vi "JKI_Sprinkler.vi"() -> ()   [LabVIEW 2016]
doc: "The sprinkler controller simulates a lawn sprinkler control system that services four \nzones: North, South, East, and West. Controls on the front panel control the zone \nselection and simulate external conditions. Indicators on the front panel indicate the zone \nthat is currently being serviced and the elapsed time for that zone."
uses:
  Controls/Zone Setup.ctl
  Controls/Zone.ctl
  Controls/Zone Indicators.ctl
panel:
  out "Zone Indicators":T1 {"Timing" format="%#.2g"}
  out "Controller Status":string
  in  "Simulation Controls":T2 {"Water Pressure Sensor (%)" scale=0.0..100.0}
  in  "Zone Setup Array":T3[](array[typedef])
  in  "Controls":T5
  # "Rain"
  # "No Rain"
  # "Continuous"
  # "Single"
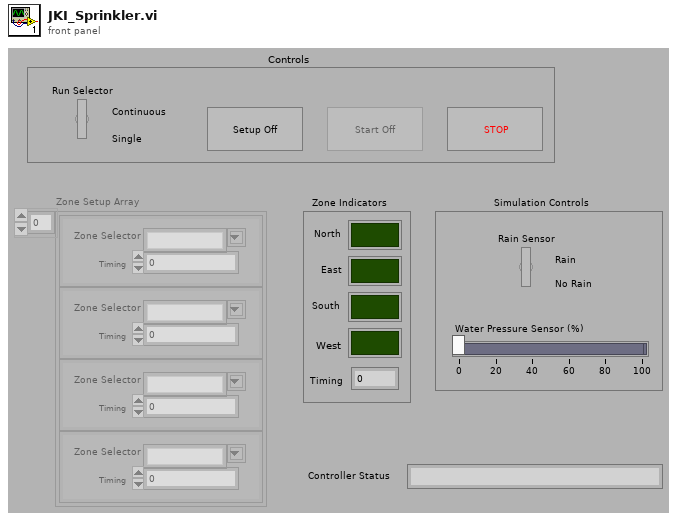
[diagram p1: front panel]
types:
  T1 = typedef "Zone Indicators.ctl" = cluster{"North":bool, "East":bool, "South":bool, "West":bool, "Timing":dbl}
  T2 = cluster{"Rain Sensor":bool, "Water Pressure Sensor (%)":dbl}
  T3 = typedef "Zone Setup.ctl" = cluster{"Zone Selector":T4, "Timing":u32}
  T4 = typedef "Zone.ctl" = string
  T5 = cluster{"Run Selector":bool, "Setup":bool, "Start":bool, "Stop":bool}
  T6 = enum32{"invalid app kind", "Development System", "Run Time System", "Student Edition", "Embedded LabVIEW", "Evaluation", "Custom"}
  T7 = enum8{"Enabled", "Disabled", "Disabled and Grayed Out"}
  T8 = enum32{"Invalid", "Standard", "Closed", "Hidden", "Minimized", "Maximized"}
  T9 = cluster{"Core":cluster{"Current VI Reference":refnum<vi>, "Close Panel on Exit?":bool}, "Your boolean":bool, "Your string data":string, "Index Zone":i32}
  T10 = cluster{"Current VI Reference":refnum<vi>, "Close Panel on Exit?":bool}
  T11 = enum16{"Always On", "Always Off", "Off While Running"}
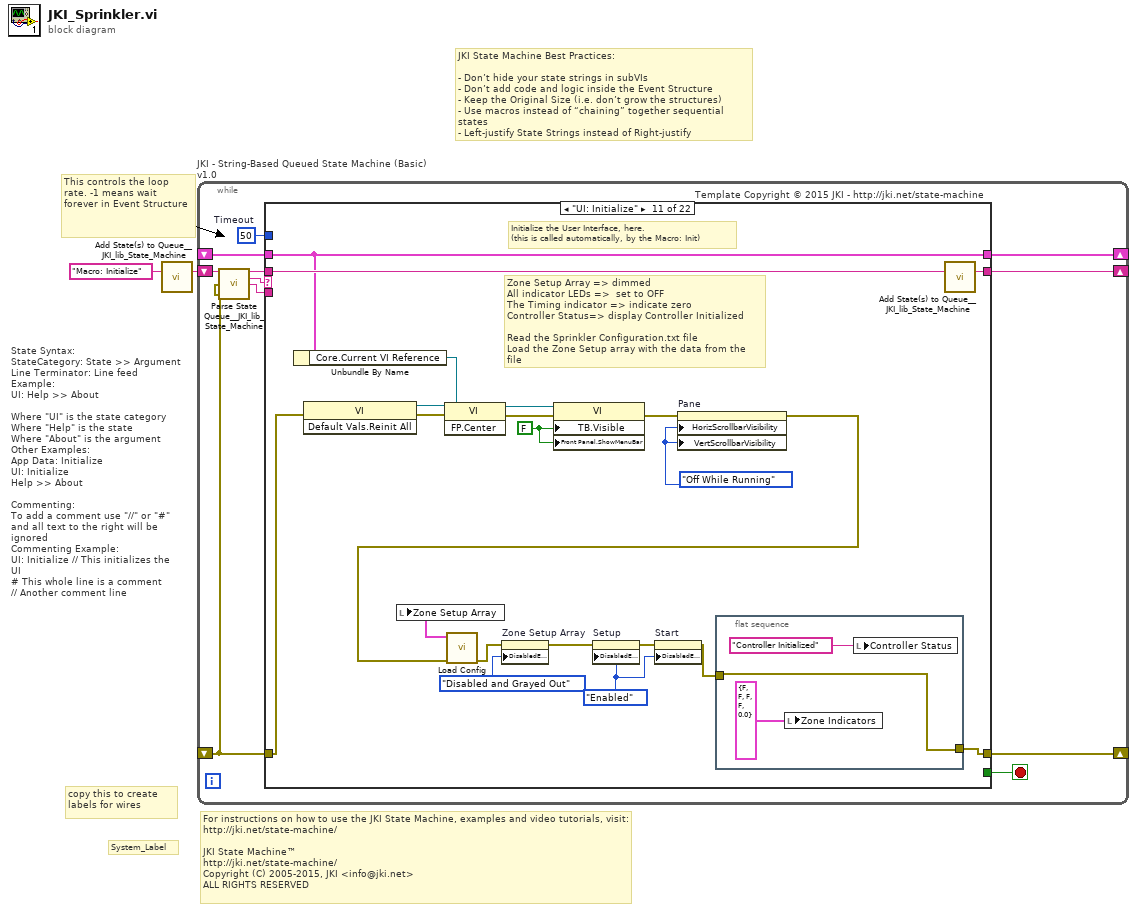
[diagram p0: block diagram]
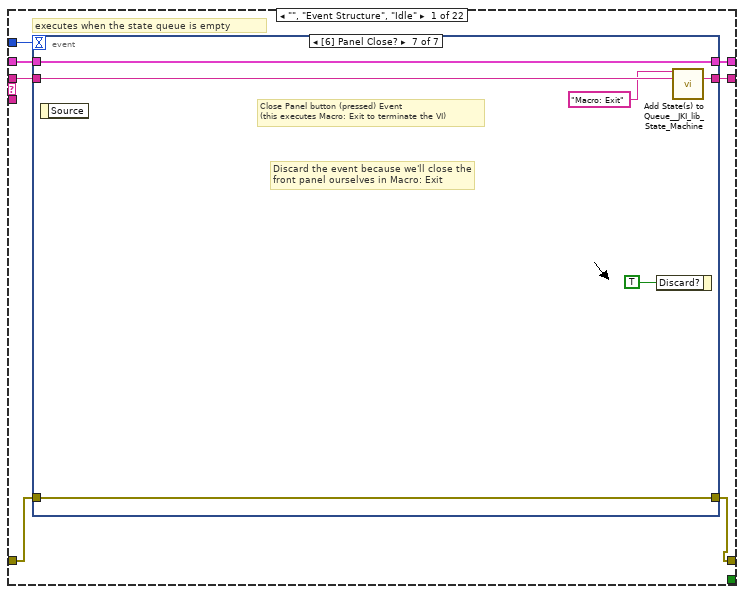
[diagram p2: hidden frame]
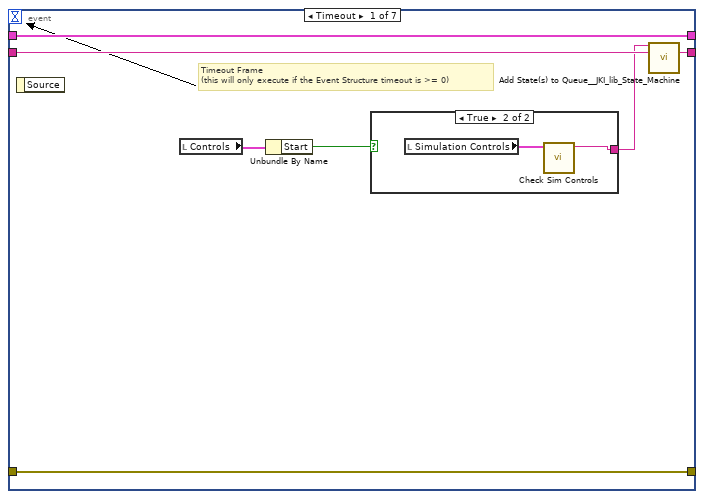
[diagram p3: hidden frame]
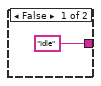
[diagram p4: hidden frame]
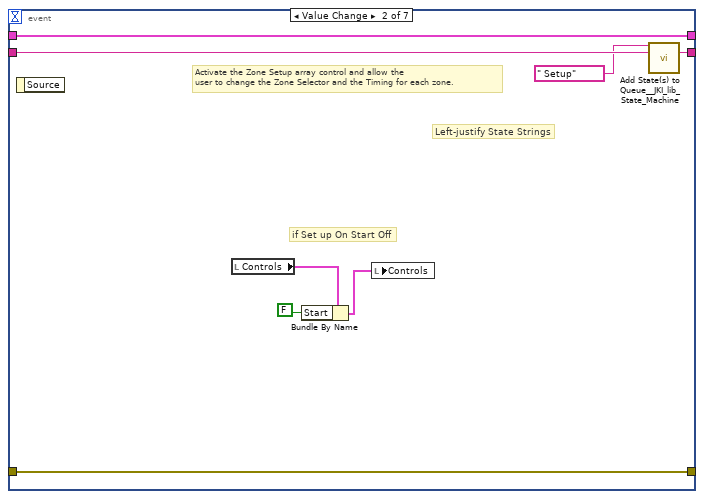
[diagram p5: hidden frame]
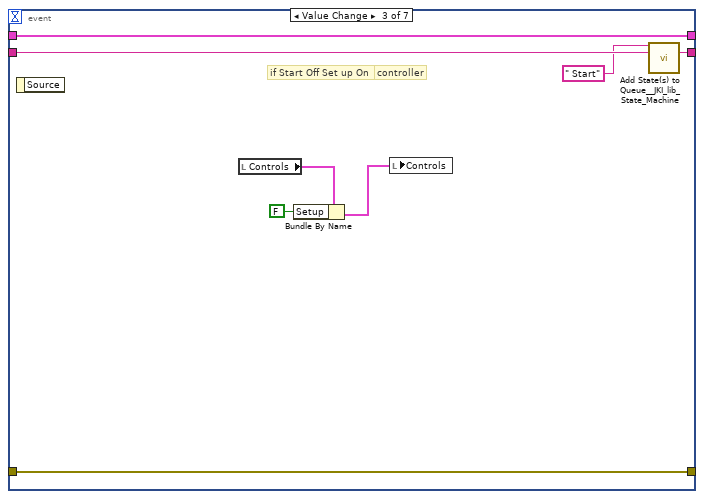
[diagram p6: hidden frame]
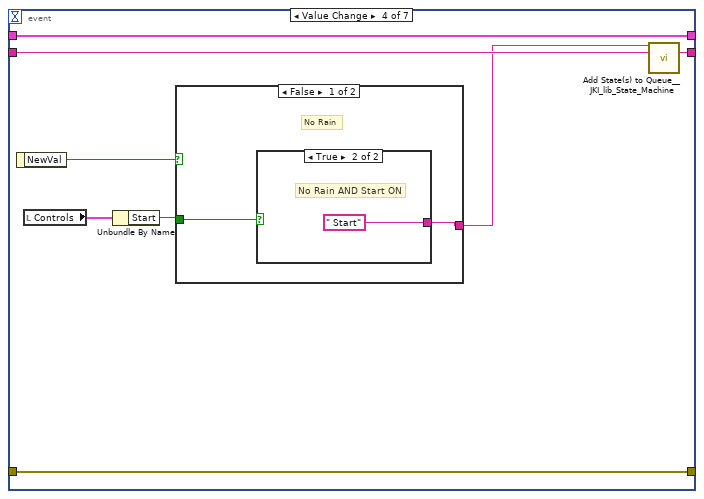
[diagram p7: hidden frame]
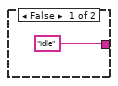
[diagram p8: hidden frame]
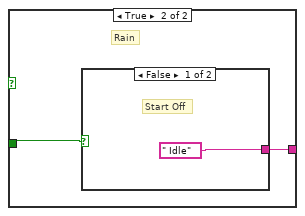
[diagram p9: hidden frame]
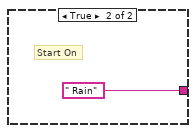
[diagram p10: hidden frame]
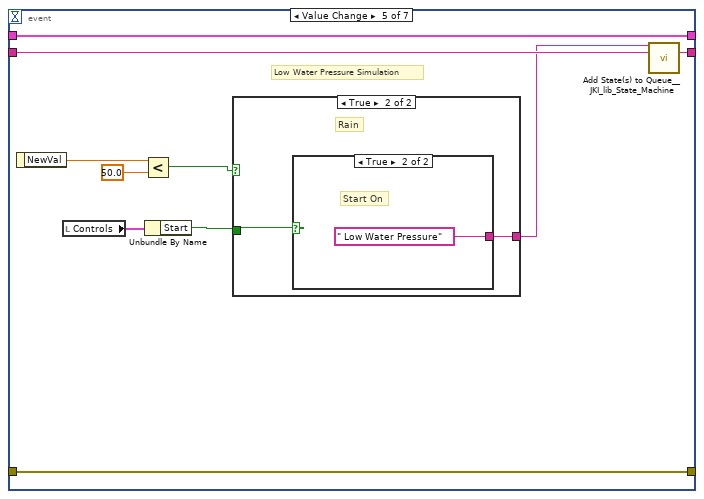
[diagram p11: hidden frame]
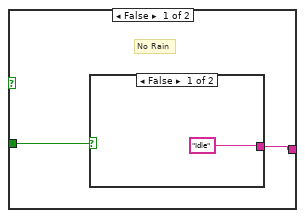
[diagram p12: hidden frame]
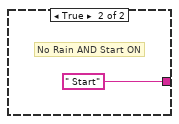
[diagram p13: hidden frame]
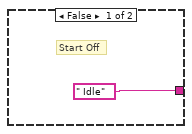
[diagram p14: hidden frame]
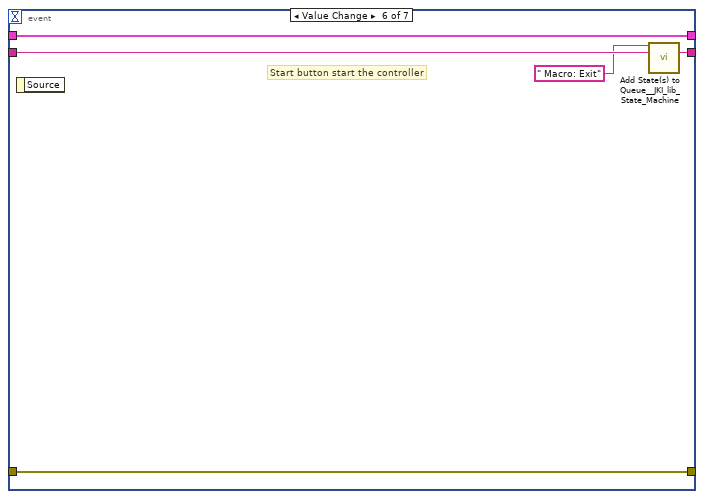
[diagram p15: hidden frame]
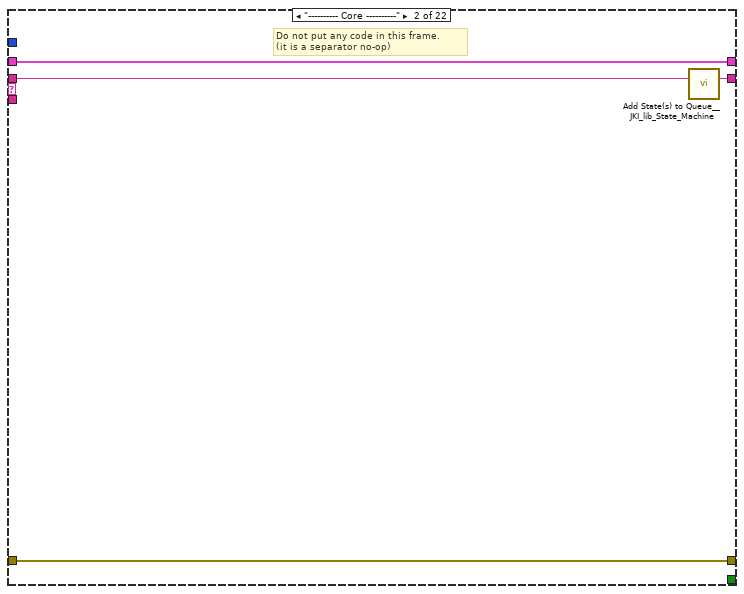
[diagram p16: hidden frame]
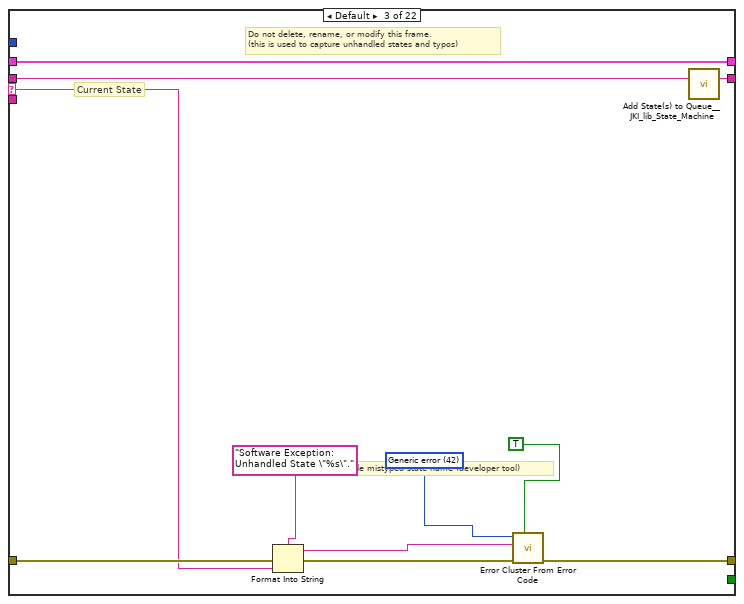
[diagram p17: hidden frame]
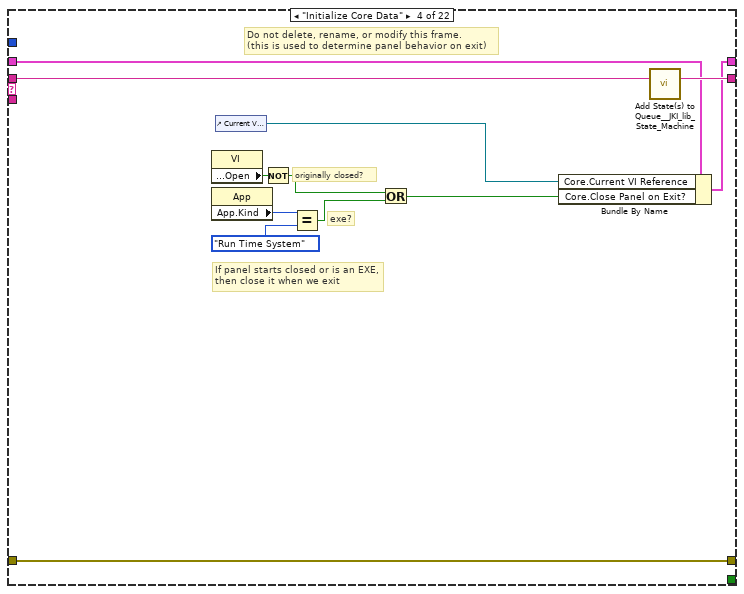
[diagram p18: hidden frame]
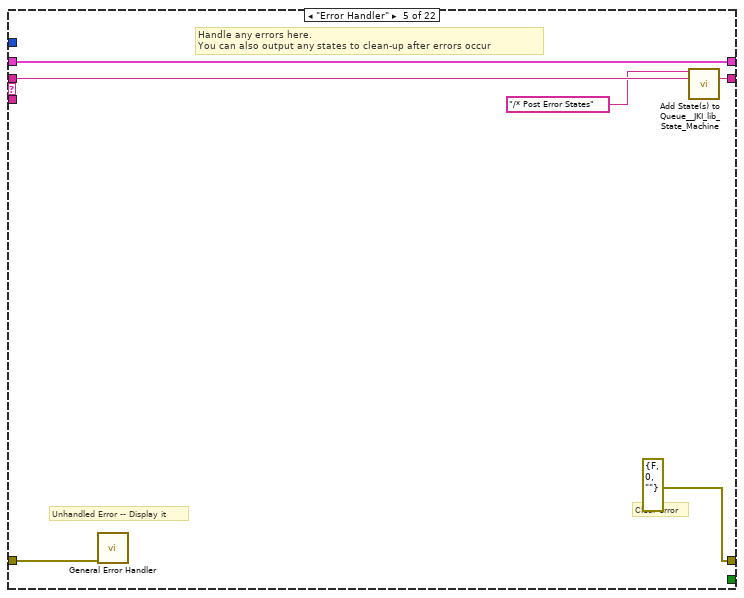
[diagram p19: hidden frame]
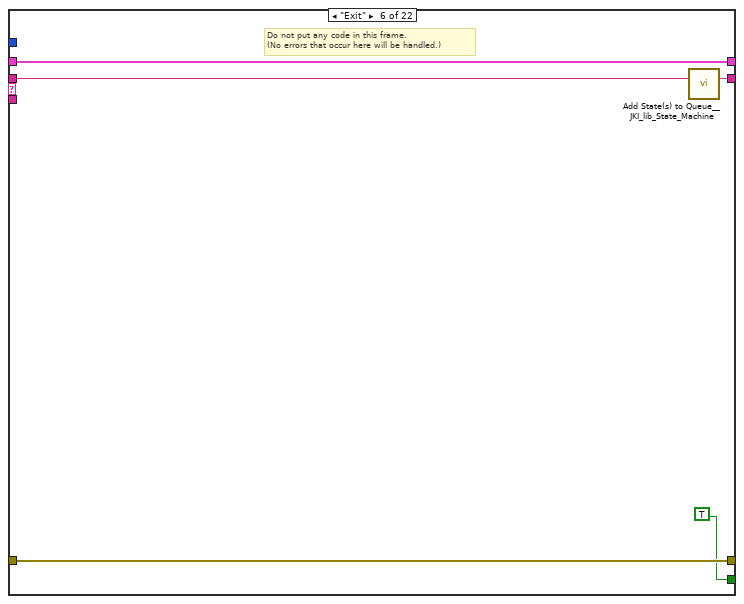
[diagram p20: hidden frame]
diagram:
  # "JKI State Machine Best Practices:\n\n- Don’t hide your state strings in subVIs\n- Don’t add code and logic inside the Event Structure\n- Keep the Original Size (i.e. don’t grow the structures)\n- Use macros instead of “chaining” together sequential states\n- Left-justify State Strings instead of Right-justify"
  # "For instructions on how to use the JKI State Machine, examples and video tutorials, visit:\nhttp://jki.net/state-machine/\n\nJKI State Machine™\nhttp://jki.net/state-machine/\nCopyright (C) 2005-2015, JKI <info@jki.net>\nALL RIGHTS RESERVED"
  # "State Syntax:\nStateCategory: State >> Argument\nLine Terminator: Line feed\nExample:\nUI: Help >> About\n\nWhere \"UI\" is the state category\nWhere \"Help\" is the state\nWhere \"About\" is the argument\nOther Examples:\nApp Data: Initialize\nUI: Initialize\nHelp >> About\n\nCommenting:\nTo add a comment use \"//\" or \"#\" and all text to the right will be ignored\nCommenting Example:\nUI: Initialize // This initializes the UI\n# This whole line is a comment\n// Another comment line"
  # "copy this to create labels for wires"
  # "This controls the loop rate. -1 means wait forever in Event Structure"
  # "System_Label"
  n1 = call <vilib>:"Add State(s) to Queue__JKI_lib_State_Machine.vi"("State(s) in (\"\")"="Macro: Initialize") -> ("States Out"=w2:string)  [unwired: 14 in]
  n2 = while "JKI - String-Based Queued State Machine (Basic) v1.0" {
    shift-right: [w6] -> _
    shift-left: _ -> [w5]
    shift-right: [w9] -> _
    shift-left: _ -> [w3]
    shift-right: [w8] -> _
    shift-left: w2 -> [w10]
    stop <- w7 stop-if-true
    w4 = 50  # Timeout
    # "Template Copyright © 2015 JKI - http://jki.net/state-machine"
    n3 = call <vilib>:"Parse State Queue__JKI_lib_State_Machine.vi"("State Queue"=w10, "Error In (no error)"=w3) -> ("Remaining States"=w12:string, "Current State"=w13:string, "Arguments"=w11:string)  [unwired: 11 in]
    n4 = case shown="\"UI: Initialize\"" w13 {
      selector: w13 -> [_ _ w96 _ _ _ _ _ _ _ _ _ _ _ _ _ _ _ _ _ _ _]
      tunnel: w12 -> [w20 w95 w100 w118 w124 w129 w133 w141 w147 w151 w171 w180 w191 w217 w222 w233 w237 w248 w264 w270 w276 w290]
      tunnel: w11 -> [_ _ _ _ _ _ _ _ _ _ _ w175 w185 _ _ _ _ _ _ _ _ _]
      tunnel: w5 -> [w18 w92 w98 w109 w121 w127 w130 _ w142 w148 w167 w178 w187 w214 w219 w230 w234 w246 w258 w268 w274 w286]
      tunnel: [w17 w93 w102 w115 errorcluster {"status"=FALSE, "code"=0, "source"=""} ("error out") w126 w131 w138 w143 w149 w153 w176 w188 w215 w220 w231 w235 w243 w260 w266 w272 w279] -> w9
      tunnel: w3 -> [w16 w93 w101 w115 w120 w126 w131 w138 w144 w149 w163 w177 w189 w215 w220 w231 w235 w245 w261 w266 w272 w281]
      tunnel: [w19 w94 w99 w117 w123 w128 w132 w140 w146 w150 w170 w179 w190 w216 w221 w232 w236 w247 w263 w269 w275 w289] -> w8
      tunnel: [_ _ _ _ _ TRUE _ _ _ _ _ _ _ _ _ _ _ _ _ _ _ _] -> w7
      tunnel: [w15 w92 w98 w116 w121 w127 w130 w139 w142 w148 w167 w178 w187 w214 w219 w230 w234 w246 w257 w268 w274 w287] -> w6
      tunnel: w4 -> [w14 _ _ _ _ _ _ _ _ _ _ _ _ _ _ _ _ _ _ _ _ _]
      frame "", "Event Structure", "Idle" {
        # "executes when the state queue is empty"
        n5 = event shown="[6] Panel Close?" {
          selector: _ -> [_ _ _ _ _ _ _]
          dyn-events: _ -> [_ _ _ _ _ _ _]
          timeout: w14 -> [_ _ _ _ _ _ _]
          tunnel: w20 -> [w27 w38 w46 w54 w72 w85 w91]
          tunnel: [w26 w37 w45 w53 w71 w84 w90] -> w19
          tunnel: w18 -> [w24 w35 w43 w51 w69 w82 w88]
          tunnel: [w25 w36 w44 w52 w70 w83 w89] -> w17
          tunnel: w16 -> [w25 w36 w44 w52 w70 w83 w89]
          tunnel: [w24 w35 w43 w51 w69 w82 w88] -> w15
          event Timeout {
            # "Timeout Frame\n(this will only execute if the Event Structure timeout is >= 0)"
            n6 = event-data() -> ()  [unwired: 1 in, 1 out]
            n7 = local read "Controls"() -> (w23:T5)
            n8 = Unbundle By Name(w23) -> ("Start"=w21:bool)
            n9 = case shown="True" w21 {
              tunnel: ["Idle" w29] -> w22
              frame False {
              }
              frame True {
                n10 = local read "Simulation Controls"() -> (w30:T2)
                n11 = call "Check Sim Controls.vi"("Simulation Controls"=w30) -> ("State"=w29:string)  [unwired: 9 in, 1 out]
              }
            }
            n12 = call <vilib>:"Add State(s) to Queue__JKI_lib_State_Machine.vi"("State(s) in Front (\"\")"=w22, "State(s) in (\"\")"=w27) -> ("States Out"=w26:string)  [unwired: 13 in]
          }
          event "Controls.Setup": Value Change {
            # "if Set up On Start Off"
            # "Left-justify State Strings"
            # "Activate the Zone Setup array control and allow the \nuser to change the Zone Selector and the Timing for each zone."
            n13 = event-data() -> ()  [unwired: 1 in, 1 out]
            n14 = local read "Controls"() -> (w33:T5)
            n15 = Bundle By Name(cluster=w33, "Start"=FALSE) -> (w32:T5)
            n16 = local write "Controls"(w32) -> ()
            n17 = call <vilib>:"Add State(s) to Queue__JKI_lib_State_Machine.vi"("State(s) in Front (\"\")"=" Setup", "State(s) in (\"\")"=w38) -> ("States Out"=w37:string)  [unwired: 13 in]
          }
          event "Controls.Start": Value Change {
            # "if Start Off Set up On"
            # "Start button start the controller"
            n18 = event-data() -> ()  [unwired: 1 in, 1 out]
            n19 = local read "Controls"() -> (w41:T5)
            n20 = Bundle By Name(cluster=w41, "Setup"=FALSE) -> (w40:T5)
            n21 = local write "Controls"(w40) -> ()
            n22 = call <vilib>:"Add State(s) to Queue__JKI_lib_State_Machine.vi"("State(s) in Front (\"\")"=" Start", "State(s) in (\"\")"=w46) -> ("States Out"=w45:string)  [unwired: 13 in]
          }
          event "Simulation Controls.Rain Sensor": Value Change {
            n23 = event-data() -> ("NewVal"=w50:bool)  [unwired: 1 in]
            n24 = local read "Controls"() -> (w49:T5)
            n25 = Unbundle By Name(w49) -> ("Start"=w48:bool)
            n26 = case shown="False" w50 {
              tunnel: w48 -> [w56 w60]
              tunnel: [w55 w59] -> w47
              frame False {
                # "No Rain"
                n27 = case shown="True" w56 {
                  tunnel: ["Idle" " Start"] -> w55
                  frame False {
                  }
                  frame True {
                    # "No Rain AND Start ON"
                  }
                }
              }
              frame True {
                # "Rain"
                n28 = case shown="False" w60 {
                  tunnel: [" Idle" " Rain"] -> w59
                  frame False {
                    # "Start Off"
                  }
                  frame True {
                    # "Start On"
                  }
                }
              }
            }
            n29 = call <vilib>:"Add State(s) to Queue__JKI_lib_State_Machine.vi"("State(s) in Front (\"\")"=w47, "State(s) in (\"\")"=w54) -> ("States Out"=w53:string)  [unwired: 13 in]
          }
          event "Simulation Controls.Water Pressure Sensor (%)": Value Change {
            # "Low Water Pressure Simulation"
            n30 = event-data() -> ("NewVal"=w68:dbl)  [unwired: 1 in]
            n31 = local read "Controls"() -> (w66:T5)
            n32 = Less?(x=w68, y=50.0) -> (x < y?=w64:bool)
            n33 = Unbundle By Name(w66) -> ("Start"=w65:bool)
            n34 = case shown="True" w64 {
              tunnel: w65 -> [w74 w78]
              tunnel: [w73 w77] -> w63
              frame False {
                # "No Rain"
                n35 = case shown="False" w74 {
                  tunnel: ["Idle" " Start"] -> w73
                  frame False {
                  }
                  frame True {
                    # "No Rain AND Start ON"
                  }
                }
              }
              frame True {
                # "Rain"
                n36 = case shown="True" w78 {
                  tunnel: [" Idle" " Low Water Pressure"] -> w77
                  frame False {
                    # "Start Off"
                  }
                  frame True {
                    # "Start On"
                  }
                }
              }
            }
            n37 = call <vilib>:"Add State(s) to Queue__JKI_lib_State_Machine.vi"("State(s) in Front (\"\")"=w63, "State(s) in (\"\")"=w72) -> ("States Out"=w71:string)  [unwired: 13 in]
          }
          event "Controls.Stop": Value Change {
            # "Start button start the controller"
            n38 = event-data() -> ()  [unwired: 1 in, 1 out]
            n39 = call <vilib>:"Add State(s) to Queue__JKI_lib_State_Machine.vi"("State(s) in Front (\"\")"=" Macro: Exit", "State(s) in (\"\")"=w85) -> ("States Out"=w84:string)  [unwired: 13 in]
          }
          event Panel Close? {
            # "Discard the event because we'll close the front panel ourselves in Macro: Exit"
            # "Close Panel button (pressed) Event\n(this executes Macro: Exit to terminate the VI)"
            n40 = event-data() -> ()  [unwired: 1 in, 1 out]
            n41 = event-data("Discard?"=TRUE) -> ()  [unwired: 1 in, 1 out]
            n42 = call <vilib>:"Add State(s) to Queue__JKI_lib_State_Machine.vi"("State(s) in Front (\"\")"="Macro: Exit", "State(s) in (\"\")"=w91) -> ("States Out"=w90:string)  [unwired: 13 in]
          }
        }
      }
      frame "---------- Core ----------" {
        # "Do not put any code in this frame.\n(it is a separator no-op)"
        n43 = call <vilib>:"Add State(s) to Queue__JKI_lib_State_Machine.vi"("State(s) in (\"\")"=w95) -> ("States Out"=w94:string)  [unwired: 14 in]
      }
      frame Default {
        w105 = 42 items=["No error", "Argument error", "Memory is full", "Out of zone", "End of file", "File already open", "Generic file I/O error", "File not found", "File permission error", "Disk is full", "Duplicate path", "Too many files open", "System feature not enabled", "Resource file not found", "Cannot add resource", "Resource not found", "Image not found", "Image memory error", "Pen does not exist", "Config type invalid", "Config token not found", "Config parse error", "Config memory error", "Bad external code format", "Bad external code offset", "External code not present", "Null window", "Destroy window error", "Null menu", "Print aborted", "Bad print record", "Print driver error", "Windows error during printing", "Memory error during printing", "Print dialog error", "Generic print error", "Invalid device refnum", "Device not found", "Device parameter error", "Device unit error", "Cannot open device", "Device call aborted", "Generic error", "Cancelled by user", "Object ID too low", "Object ID too high", "Object not in heap", "Unknown heap", "Unknown object (invalid DefProc)", "Unknown object (DefProc not in table)", "Message out of range", "Invalid (null) method", "Unknown message", "Manager call not supported", "Bad address", "Network operation in progress", "Network operation timed out", "Connection is busy", "Network attribute not supported", "Network error", "Address in use", "System out of memory", "Connection aborted", "Connection refused", "Not connected", "Already connected", "Connection closed", "Initialization error (interapplication manager)", "Bad occurrence", "Wait on unbound occurrence handler", "Occurrence queue overflow", "Datalog type conflict", "Unused", "Unrecognized type (interapplication manager)", "Memory corrupt", "Failed to make temporary DLL", "Old CIN version", "Drag socket not found", "Failed to load drop-object", "Failed to register OLE object", "Failed to release OLE object", "Format specifier type mismatch", "Unknown format specifier", "Too few format specifiers", "Too many format specifiers", "Scan failed", "Newer CIN version", "Error converting to variant", "Runtime menu error", "Password tampered", "Variant attribute not found", "Incompatible variant data type", "Event data is not available", "Event Store is not present", "Occurrence is not found", "Event Queue is not created", "Event info is not available", "Refnum passed is NULL", "Error retrieving Class GUID", "Error retrieving CoClass GUID", "Error retrieving TypeLib GUID.", "Bad built application magic bytes.", "Specific driver is different from the specific driver associated with the Logical Name.", "There is no session opened to the class driver.", "Max Error", "MAX - Error with config objects", "MAX - Error loading configuration", "MAX - Group not supported"]
        # "Current State"
        # "Do not delete, rename, or modify this frame.\n(this is used to capture unhandled states and typos)"
        # "Handle mistyped state name (developer tool)"
        n44 = Format Into String(format string="Software Exception: Unhandled State \"%s\"." ("message"), error in=w101, w96) -> (resulting string=w104:string, error out=w103:errorcluster)  [unwired: 1 in]
        n45 = call <vilib>:"Error Cluster From Error Code.vi"("show call chain? (False)"=TRUE, "error in (no error)"=w103, "error message (\"\")"=w104, "error code (0)"=w105) -> ("error out"=w102:errorcluster)  [unwired: 5 in]
        n46 = call <vilib>:"Add State(s) to Queue__JKI_lib_State_Machine.vi"("State(s) in (\"\")"=w100) -> ("States Out"=w99:string)  [unwired: 14 in]
      }
      frame "Initialize Core Data" {
        # "Do not delete, rename, or modify this frame.\n(this is used to determine panel behavior on exit)"
        # "originally closed?"
        # "exe?"
        # "If panel starts closed or is an EXE, then close it when we exit"
        n47 = property class="VI"() -> ("Front Panel.Open"=w114:bool)  [unwired: 2 in, 2 out]
        n48 = property class="App"() -> ("App.Kind"=w113:T6)  [unwired: 2 in, 2 out]
        n49 = control-ref of="Current VI Reference"() -> (w107:refnum<vi>)
        n50 = Not(x=w114) -> (.not. x?=w111:bool)
        n51 = Equal?(x=w113, y=T6."Run Time System" ("Application:Kind")) -> (x = y?=w110:bool)
        n52 = Or(x=w111, y=w110) -> (x .or. y?=w108:bool)
        n53 = Bundle By Name(cluster=w109, "Core.Current VI Reference"=w107, "Core.Close Panel on Exit?"=w108) -> (w116:T9)
        n54 = call <vilib>:"Add State(s) to Queue__JKI_lib_State_Machine.vi"("State(s) in (\"\")"=w118) -> ("States Out"=w117:string)  [unwired: 14 in]
      }
      frame "Error Handler" {
        # "Unhandled Error -- Display it"
        # "Handle any errors here.\nYou can also output any states to clean-up after errors occur"
        # "Clear error"
        n55 = call <vilib>:"General Error Handler.vi"("error in (no error)"=w120) -> ()  [unwired: 10 in, 5 out]
        n56 = call <vilib>:"Add State(s) to Queue__JKI_lib_State_Machine.vi"("State(s) in Front (\"\")"="/* Post Error States", "State(s) in (\"\")"=w124) -> ("States Out"=w123:string)  [unwired: 13 in]
      }
      frame "Exit" {
        # "Do not put any code in this frame.\n(No errors that occur here will be handled.)"
        n57 = call <vilib>:"Add State(s) to Queue__JKI_lib_State_Machine.vi"("State(s) in (\"\")"=w129) -> ("States Out"=w128:string)  [unwired: 14 in]
      }
      frame "---------- Data ----------" {
        # "Do not put any code in this frame.\n(It is a separator no-op. You can make a copy of this frame to create a new Data frame)"
        n58 = call <vilib>:"Add State(s) to Queue__JKI_lib_State_Machine.vi"("State(s) in (\"\")"=w133) -> ("States Out"=w132:string)  [unwired: 14 in]
      }
      frame "Data: Initialize" {
        w134 = TRUE  # Your boolean
        w135 = 0  # Index Zone
        w136 = T10 {"Current VI Reference"=refnum, "Close Panel on Exit?"=FALSE}  # Core
        w137 = ""  # Your string data
        # "do not delete - used by framework"
        # "Expand Bundle to add new data elements to shift register data."
        # "Data names and types of shift register data are defined by this bundle."
        # "Initialize the shift-register data, here.\n(data names are defined by what you wire into the bundle function)"
        n59 = Bundle("Core"=w136, "Your boolean"=w134, "Your string data"=w137, "Index Zone"=w135) -> (w139:T9)  [unwired: 1 in]
        n60 = call <vilib>:"Add State(s) to Queue__JKI_lib_State_Machine.vi"("State(s) in (\"\")"=w141) -> ("States Out"=w140:string)  [unwired: 14 in]
      }
      frame "Data: Cleanup" {
        # "Cleanup any data and references, here.\n(this is called automatically, by the Macro: Exit)"
        n61 = Unbundle By Name(w142) -> ("Core.Current VI Reference"=w145:refnum<vi>)
        n62 = Close Reference(reference=w145, error in (no error)=w144) -> (error out=w143:errorcluster)
        n63 = call <vilib>:"Add State(s) to Queue__JKI_lib_State_Machine.vi"("State(s) in (\"\")"=w147) -> ("States Out"=w146:string)  [unwired: 14 in]
      }
      frame "---------- UI ----------" {
        # "Do not put any code in this frame.\n(It is a separator no-op. You can make a copy of this frame to create a new UI frame)"
        n64 = call <vilib>:"Add State(s) to Queue__JKI_lib_State_Machine.vi"("State(s) in (\"\")"=w151) -> ("States Out"=w150:string)  [unwired: 14 in]
      }
      frame "UI: Initialize" {
        w152 = T11."Off While Running" ("Horizontal Scrollbar Visibility")
        w164 = FALSE ("Tool Bar:Visible")
        w156 = T7."Enabled" ("Disabled")
        # "Zone Setup Array => dimmed \nAll indicator LEDs =>  set to OFF \nThe Timing indicator => indicate zero  \nController Status=> display Controller Initialized\n\nRead the Sprinkler Configuration.txt file\nLoad the Zone Setup array with the data from the file"
        # "Initialize the User Interface, here.\n(this is called automatically, by the Macro: Init)"
        n65 = Unbundle By Name(w167) -> ("Core.Current VI Reference"=w166:refnum<vi>)
        n66 = invoke class="VI" method="Default Vals.Reinit All"(reference=w166, error in=w163) -> (error out=w162:errorcluster)  [unwired: 1 in, 2 out]
        n67 = invoke class="VI" method="FP.Center"(reference=w166, error in=w162) -> (reference out=w165:refnum<vi>, error out=w161:errorcluster)  [unwired: 1 in, 1 out]
        n68 = property class="VI"(reference=w165, error in=w161, "TB.Visible"=w164, "Front Panel.ShowMenuBar"=w164) -> (error out=w160:errorcluster)  [unwired: 1 out]
        n69 = property on="Pane" class="Pane"(error in=w160, "HorizScrollbarVisibility"=w152, "VertScrollbarVisibility"=w152) -> (error out=w159:errorcluster)  [unwired: 1 in, 1 out]
        n70 = call "Load Config.vi"("error in"=w159) -> ("error out"=w158:errorcluster, "Zone Setup Array"=w168:T3[])  [unwired: 9 in]
        n71 = local write "Zone Setup Array"(w168) -> ()
        n72 = property on="Zone Setup Array" class="Arr (strict)"(error in=w158, "DisabledEnum"=T7."Disabled and Grayed Out" ("Disabled")) -> (error out=w157:errorcluster)  [unwired: 1 in, 1 out]
        n73 = property on="Setup" class="Bool (strict)"(error in=w157, "DisabledEnum"=w156) -> (error out=w155:errorcluster)  [unwired: 1 in, 1 out]
        n74 = property on="Start" class="Bool (strict)"(error in=w155, "DisabledEnum"=w156) -> (error out=w154:errorcluster)  [unwired: 1 in, 1 out]
        n75 = flat-sequence {
          tunnel: w154 -> [w172]
          tunnel: [w172] -> w153
          frame #0 {
            n76 = local write "Zone Indicators"(T1 {"North"=FALSE, "East"=FALSE, "South"=FALSE, "West"=FALSE, "Timing"=0.0} ("Zone Indicators")) -> ()
            n77 = local write "Controller Status"("Controller Initialized") -> ()
          }
        }
        n78 = call <vilib>:"Add State(s) to Queue__JKI_lib_State_Machine.vi"("State(s) in (\"\")"=w171) -> ("States Out"=w170:string)  [unwired: 14 in]
      }
      frame "UI: Cursor Set" {
        # "Argument"
        # "Set and Unset Cursor Busy.\n(Usage: \"UI: Cursor Set >> Busy|Idle\")"
        n79 = case shown="\"Idle\", Default" w175 {
          tunnel: w177 -> [w182 w184]
          tunnel: [w181 w183] -> w176
          frame "Idle", Default {
            n80 = call <vilib>:"Unset Busy.vi"("error in (no error)"=w182) -> ("error out"=w181:errorcluster)  [unwired: 10 in]
          }
          frame "Busy" {
            n81 = call <vilib>:"Set Busy.vi"("error in (no error)"=w184) -> ("error out"=w183:errorcluster)  [unwired: 9 in, 1 out]
          }
        }
        n82 = call <vilib>:"Add State(s) to Queue__JKI_lib_State_Machine.vi"("State(s) in (\"\")"=w180) -> ("States Out"=w179:string)  [unwired: 14 in]
      }
      frame "UI: Front Panel State" {
        # "Argument"
        # "Set Front Panel Open or Closed\n(Usage: \"UI: Front Panel State >> Open|Close\")"
        n83 = Unbundle By Name(w187) -> ("Core.Current VI Reference"=w186:refnum<vi>)
        n84 = case shown="\"Open\", Default" w185 {
          tunnel: w189 -> [w195 w208]
          tunnel: [w197 w209] -> w188
          tunnel: w186 -> [w196 w206]
          frame "Open", Default {
            n85 = property class="VI"(reference=w196, error in=w195) -> (reference out=w193:refnum<vi>, error out=w194:errorcluster, "Front Panel.Open"=w192:bool)
            n86 = case shown="True" w192 {
              tunnel: [w200 w203] -> w197
              tunnel: w194 -> [w199 w203]
              tunnel: w193 -> [w198 _]
              frame False {
                n87 = invoke class="VI" method="FP.Open"(reference=w198, error in=w199, "Activate"=TRUE, "State"=T8."Standard") -> (error out=w200:errorcluster)  [unwired: 1 in, 4 out]
              }
              frame True {
              }
            }
          }
          frame "Close" {
            n88 = property class="VI"(reference=w206, error in=w208) -> (reference out=w205:refnum<vi>, error out=w207:errorcluster, "Front Panel.Open"=w204:bool)
            n89 = case shown="True" w204 {
              tunnel: [w210 w213] -> w209
              tunnel: w207 -> [w210 w212]
              tunnel: w205 -> [_ w211]
              frame False {
              }
              frame True {
                n90 = invoke class="VI" method="FP.Close"(reference=w211, error in=w212) -> (error out=w213:errorcluster)  [unwired: 1 in, 2 out]
              }
            }
          }
        }
        n91 = call <vilib>:"Add State(s) to Queue__JKI_lib_State_Machine.vi"("State(s) in (\"\")"=w191) -> ("States Out"=w190:string)  [unwired: 14 in]
      }
      frame "---------- Macro ----------" {
        # "Do not put any code in this frame.\n(It is a separator no-op. You can make a copy of this frame to create a new Macro frame)"
        n92 = call <vilib>:"Add State(s) to Queue__JKI_lib_State_Machine.vi"("State(s) in (\"\")"=w217) -> ("States Out"=w216:string)  [unwired: 14 in]
      }
      frame "Macro: Initialize" {
        w218 = "Data: Initialize\nInitialize Core Data\nUI: Initialize\nUI: Front Panel State >> Open"  # Data: Initialize Initialize Core Data UI: Initialize UI: Front Panel State >> Open
        # "Initialization Macro\n(This is called once, when the VI starts)"
        n93 = call <vilib>:"Add State(s) to Queue__JKI_lib_State_Machine.vi"("State(s) in Front (\"\")"=w218, "State(s) in (\"\")"=w222) -> ("States Out"=w221:string)  [unwired: 13 in]
      }
      frame "Macro: Exit" {
        # "Stop servicing the zones \nDisplay Stopped in the Controller Status indicator \nStop the application"
        # "Exit Macro\n(This is called once, when the VI exits)"
        n94 = Unbundle By Name(w230) -> ("Core.Close Panel on Exit?"=w229:bool)
        n95 = local write "Controller Status"("Stopped" ("Controller Status")) -> ()
        n96 = Select(t="UI: Front Panel State >> Close", s=w229, f="") -> (s? t:f=w226:string)
        n97 = call <vilib>:"Add State(s) to Queue__JKI_lib_State_Machine.vi"("State(s) in (\"\")"=w226, "State(s) at Back (\"\")"="Data: Cleanup\nExit") -> ("States Out"=w224:string)  [unwired: 13 in]
        n98 = call <vilib>:"Add State(s) to Queue__JKI_lib_State_Machine.vi"("State(s) in Front (\"\")"=w224, "State(s) in (\"\")"=w233) -> ("States Out"=w232:string)  [unwired: 13 in]
      }
      frame "---------- Sprinkler ----------" {
        # "Template Separator\n(You can make a copy of, or modify, this frame)"
        n99 = call <vilib>:"Add State(s) to Queue__JKI_lib_State_Machine.vi"("State(s) in (\"\")"=w237) -> ("States Out"=w236:string)  [unwired: 14 in]
      }
      frame "Setup" {
        w238 = T7."Enabled" ("Disabled")
        # "Activate the Zone Setup array control and allow the \nuser to change the Zone Selector and the Timing for each zone.\n\n The Controller Status display Setup Mode"
        n100 = property on="Zone Setup Array" class="Arr (strict)"(error in=w245, "DisabledEnum"=w238) -> (error out=w239:errorcluster)  [unwired: 1 in, 1 out]
        n101 = property on="Start" class="Bool (strict)"(error in=w239, "DisabledEnum"=w238) -> (error out=w240:errorcluster)  [unwired: 1 in, 1 out]
        n102 = property on="Setup" class="Bool (strict)"(error in=w240, "DisabledEnum"=T7."Disabled and Grayed Out" ("Disabled")) -> (error out=w243:errorcluster)  [unwired: 1 in, 1 out]
        n103 = local write "Zone Indicators"(T1 {"North"=FALSE, "East"=FALSE, "South"=FALSE, "West"=FALSE, "Timing"=0.0} ("Zone Indicators")) -> ()
        n104 = local write "Controller Status"("Setup Mode" ("Controller Status")) -> ()
        n105 = call <vilib>:"Add State(s) to Queue__JKI_lib_State_Machine.vi"("State(s) in (\"\")"=w248) -> ("States Out"=w247:string)  [unwired: 14 in]
      }
      frame "Start" {
        w252 = T7."Disabled and Grayed Out" ("Disabled")
        # "Rester timer\nbefore running"
        # "Reset Inex Zone"
        # "Output:\n- Low Water Pressure\n- Rain\n- Running\n- Stop"
        # "- Dim the Zone Setup array control. \n\n- Check the Water Pressure Sensor simulation control. If the water pressure is \nbelow 50 %, the Controller Status should display Low Water Pressure. If \nthe water pressure is restored to a value greater than 50 %, the controller \nshould start operating. \n\n- Run the controller in the mode selected by the Run Selector switch.  \n\n- Display Running in the Controller Status indicator."
        n106 = property on="Zone Setup Array" class="Arr (strict)"(error in=w261, "DisabledEnum"=w252) -> (error out=w254:errorcluster)  [unwired: 1 in, 1 out]
        n107 = property on="Start" class="Bool (strict)"(error in=w254, "DisabledEnum"=w252) -> (error out=w255:errorcluster)  [unwired: 1 in, 1 out]
        n108 = property on="Setup" class="Bool (strict)"(error in=w255, "DisabledEnum"=T7."Enabled" ("Disabled")) -> (error out=w251:errorcluster)  [unwired: 1 in, 1 out]
        n109 = Bundle By Name(cluster=w258, "Index Zone"=0) -> (w257:T9)
        n110 = call "Timer.vi"("error constant"=w251, "Reset"=TRUE) -> ("error constant 2"=w250:errorcluster)  [unwired: 7 in, 2 out]
        n111 = local read "Simulation Controls"() -> (w262:T2)
        n112 = call "Check Sim Controls.vi"("error in (no error)"=w250, "Simulation Controls"=w262) -> ("error out"=w260:errorcluster, "State"=w259:string)  [unwired: 8 in]
        n113 = call <vilib>:"Add State(s) to Queue__JKI_lib_State_Machine.vi"("State(s) in Front (\"\")"=w259, "State(s) in (\"\")"=w264) -> ("States Out"=w263:string)  [unwired: 13 in]
      }
      frame "Low Water Pressure" {
        # "Stay in state until water pressure go above 50%"
        n114 = local write "Controller Status"("Low Water Pressure" ("Controller Status")) -> ()
        n115 = local write "Zone Indicators"(T1 {"North"=FALSE, "East"=FALSE, "South"=FALSE, "West"=FALSE, "Timing"=0.0} ("Zone Indicators")) -> ()
        n116 = call <vilib>:"Add State(s) to Queue__JKI_lib_State_Machine.vi"("State(s) in (\"\")"=w270) -> ("States Out"=w269:string)  [unwired: 14 in]
      }
      frame "Rain" {
        # "Stay in state until rain stop"
        n117 = local write "Controller Status"("Rain" ("Controller Status")) -> ()
        n118 = local write "Zone Indicators"(T1 {"North"=FALSE, "East"=FALSE, "South"=FALSE, "West"=FALSE, "Timing"=0.0} ("Zone Indicators")) -> ()
        n119 = call <vilib>:"Add State(s) to Queue__JKI_lib_State_Machine.vi"("State(s) in (\"\")"=w276) -> ("States Out"=w275:string)  [unwired: 14 in]
      }
      frame "Running" {
        n120 = Unbundle By Name(w286) -> ("Index Zone"=w285:i32)
        n121 = call "Update.vi"("error constant"=w281, "Controls"="Controls", "Zone Setup Array"="Zone Setup Array", "Index Zone in"=w285) -> ("error constant 2"=w280:errorcluster, "Zone Indicators"=→"Zone Indicators":T1, "Index Zone out"=w282:i32)  [unwired: 5 in]
        n122 = Bundle By Name(cluster=w286, "Index Zone"=w282) -> (w287:T9)
        n123 = call "Check Sim Controls.vi"("error in (no error)"=w280, "Simulation Controls"="Simulation Controls") -> ("error out"=w279:errorcluster)  [unwired: 8 in, 1 out]
        n124 = call <vilib>:"Add State(s) to Queue__JKI_lib_State_Machine.vi"("State(s) in (\"\")"=w290) -> ("States Out"=w289:string)  [unwired: 14 in]
        "Controller Status" <- "Running" ("Controller Status")
      }
    }
  }
